vi "Terminal Checker.vi"(8 "error in (no error)":errorcluster, 11 "control reference":refnum<vi>) -> (0 "error out":errorcluster, 3 "is connected?":bool)   [LabVIEW 2013]
doc: "This VI is designed to be called in a VI that is a sub VI of a higher-level VI. A control reference from the higher-level subVI is passed into this VI, and this VI will return true if the connector pane terminal which said control reference belongs to is connected, and false if is is disconnected."
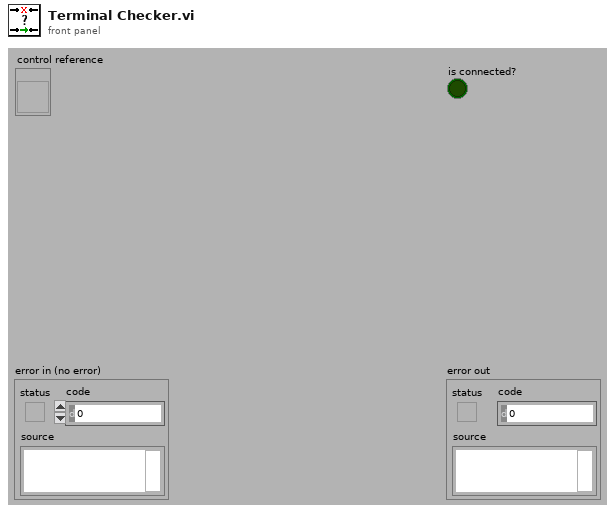
[diagram p1: front panel]
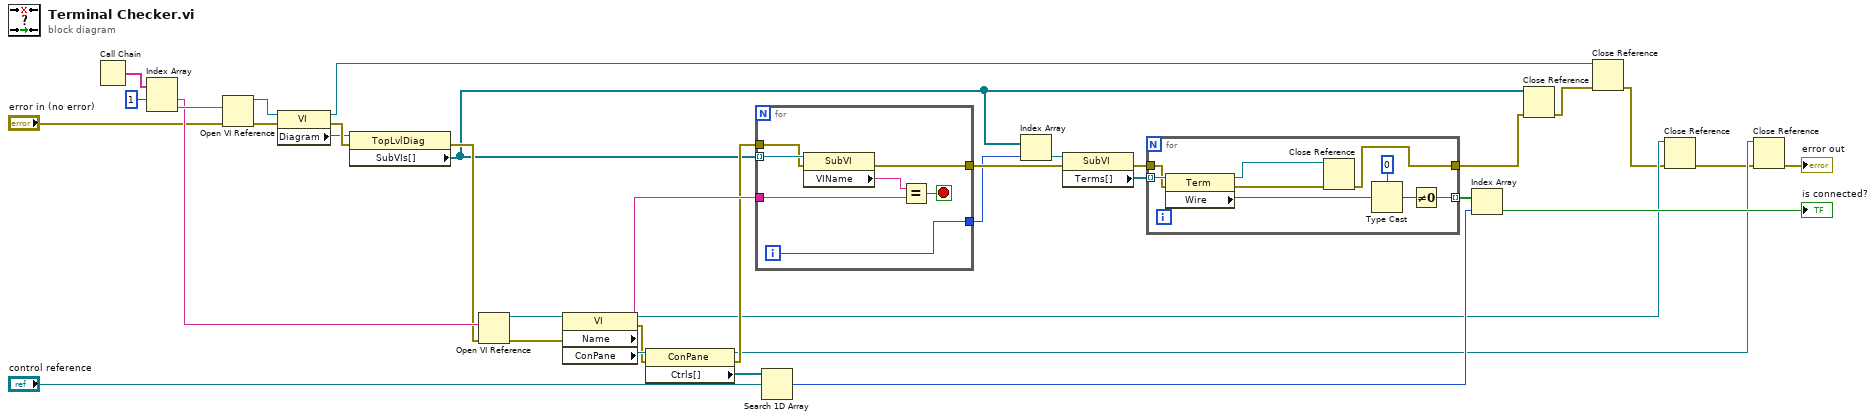
[diagram p0: block diagram]
diagram:
  n1 = Call Chain() -> (call chain=w22:string[])
  n2 = Index Array(array=w22, index #1=1 ("index")) -> (element #1=w19:string, element #2=w20:string)  [unwired: 1 in]
  n3 = Open VI Reference(vi path=w20, error in (no error)="error in (no error)") -> (vi reference=w24:refnum<vi>, error out=w25:errorcluster)  [unwired: 4 in]
  n4 = property class="VI"(reference=w24, error in=w25) -> (reference out=w6:refnum<vi>, error out=w27:errorcluster, "Diagram"=w26:refnum<vi>)
  n5 = property class="TopLvlDiag"(reference=w26, error in=w27) -> (error out=w15:errorcluster, "SubVIs[]"=w8:refnum<vi>[])  [unwired: 1 out]
  n6 = Open VI Reference(vi path=w19, error in (no error)=w15) -> (vi reference=w18:refnum<vi>, error out=w14:errorcluster)  [unwired: 4 in]
  n7 = property class="VI"(reference=w18, error in=w14) -> (reference out=w5:refnum<vi>, error out=w12:errorcluster, "Name"=w28:string, "ConPane"=w13:refnum<vi>)
  n8 = property class="ConPane"(reference=w13, error in=w12) -> (reference out=w4:refnum<vi>, error out=w11:errorcluster, "Ctrls[]"=w21:refnum<vi>[])
  n9 = for {
    tunnel: w8 -> [w42] mode=indexing
    tunnel: w28 -> [w40]
    tunnel: [w38] -> w29
    tunnel: w11 -> [w37]
    tunnel: [w36] -> w31
    i -> [w38]
    stop <- w39 stop-if-true
    n10 = property class="SubVI"(reference=w42, error in=w37) -> (error out=w36:errorcluster, "VIName"=w41:string)  [unwired: 1 out]
    n11 = Equal?(x=w41, y=w40) -> (x = y?=w39:bool)
  }
  n12 = Search 1D Array(1D array=w21, element="control reference") -> (index of element=w34:i32)  [unwired: 1 in]
  n13 = Index Array(array=w8, index=w29) -> (element=w30:refnum<vi>)
  n14 = property class="SubVI"(reference=w30, error in=w31) -> (error out=w10:errorcluster, "Terms[]"=w32:refnum<vi>[])  [unwired: 1 out]
  n15 = for {
    tunnel: w32 -> [w51] mode=indexing
    tunnel: [w47] -> w33 mode=indexing
    tunnel: w10 -> [w46]
    tunnel: [w43] -> w9
    n16 = property class="Term"(reference=w51, error in=w46) -> (reference out=w44:refnum<vi>, error out=w45:errorcluster, "Wire"=w49:refnum<vi>)
    n17 = Close Reference(reference=w44, error in (no error)=w45) -> (error out=w43:errorcluster)
    n18 = Type Cast(type=0, x=w49) -> (*(type *) &x=w48:i32)
    n19 = Not Equal To 0?(x=w48) -> (x != 0?=w47:bool)
  }
  n20 = Index Array(array=w33, index=w34) -> (element=→"is connected?":bool)
  n21 = Close Reference(reference=w8, error in (no error)=w9) -> (error out=w7:errorcluster)
  n22 = Close Reference(reference=w6, error in (no error)=w7) -> (error out=w3:errorcluster)
  n23 = Close Reference(reference=w5, error in (no error)=w3) -> (error out=w2:errorcluster)
  n24 = Close Reference(reference=w4, error in (no error)=w2) -> (error out=→"error out":errorcluster)
